vi "Save File Create Configuration Path.vi"(6 "File Type (.ini)":string=".ini", 8 "Error In":errorcluster, 9 "Configuration Name":string="Newfi Configuration_", 10 "Station ID":string, 11 "Tool Base Path":path) -> (0 "Error Out":errorcluster, 3 "New Configuration File Path":path)   [LabVIEW 2019]
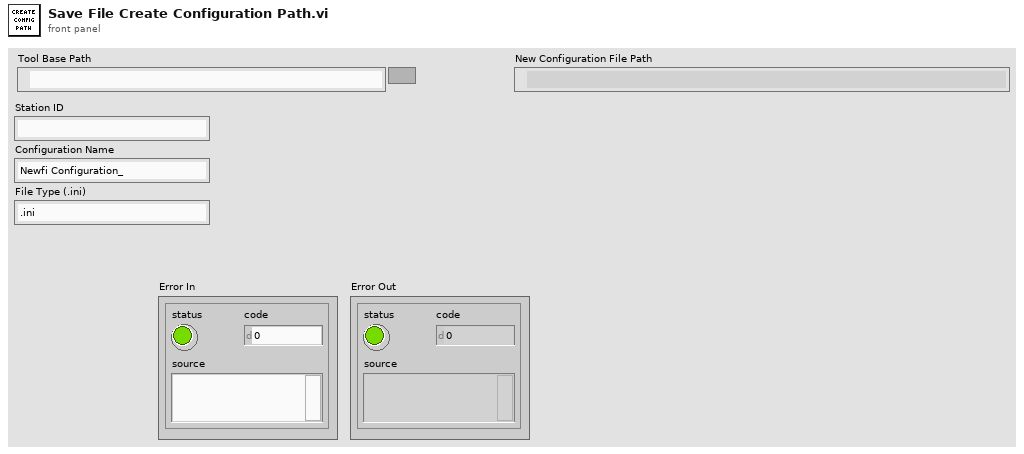
[diagram p1: front panel]
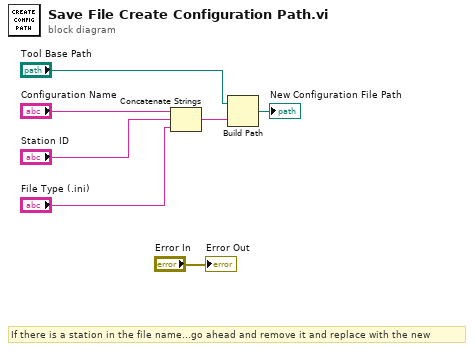
[diagram p0: block diagram]
diagram:
  # "If there is a station in the file name...go ahead and remove it and replace with the new"
  n1 = Concatenate Strings("Configuration Name", "Station ID", "File Type (.ini)") -> (w6:string)
  n2 = Build Path(base path="Tool Base Path", name or relative path=w6) -> (appended path=→"New Configuration File Path":path)
  "Error Out" <- "Error In"
